vi "Launch Subordinate.vi"(6 "Position":T1, 8 "error in":errorcluster, 9 "Panel Definiton":T3, 10 "Identifier":string, 11 "Base Software in":refnum<class "Base Software.lvclass">) -> (0 "error out":errorcluster, 2 "Subordinate":T2, 3 "Base Software out":refnum<class "Base Software.lvclass">)   [LabVIEW 2019, in "Base Software.lvlib" / "Main.lvlib" / "Base Software.lvclass"]
uses:
  Project/Base Software.lvclass
  builds/Engine/Panel Manager.lvlibp/Panel Actor/Panel Actor.lvclass
  C:/Users/Public/Documents/Development/builds/Engine/Monitored Actor.lvlibp/Monitored Actor/Monitored Actor/Monitored Actor.lvclass
  builds/Engine/Panel.lvlibp/Panel/Panel.lvclass
  Custom Controls/Subordinate.ctl
  builds/Engine/Actor Framework.lvlibp/1abvi3w/vi.lib/ActorFramework/Message Enqueuer/Message Enqueuer.lvclass
  Custom Controls/Panel_Positions.ctl
  C:/Users/Public/Documents/Development/builds/Engine/Panel Manager.lvlibp/Panel Actor/Panel Actor.lvclass
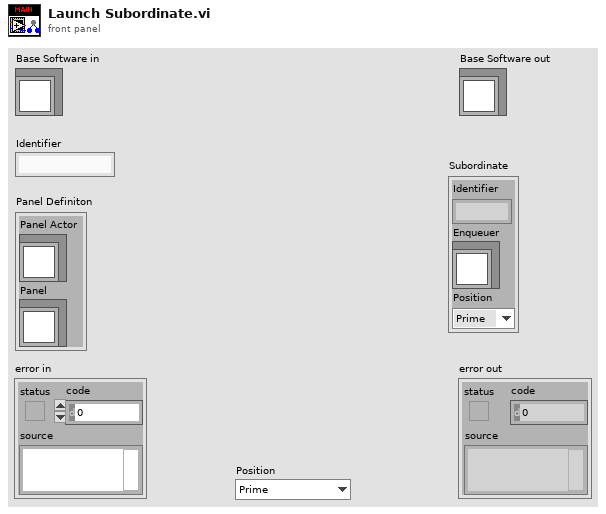
[diagram p1: front panel]
types:
  T1 = typedef "Base Software.lvlib/Main.lvlib/Base Software.lvclass/Panel_Positions.ctl" = enum16{"Prime", "Right", "Bottom", "Left", "Mission"}
  T2 = typedef "Base Software.lvlib/Main.lvlib/Base Software.lvclass/Subordinate.ctl" = cluster{"Identifier":string, "Enqueuer":refnum<class "Message Enqueuer.lvclass">, "Position":T1}
  T3 = cluster{"Panel Actor":refnum<class "Panel Actor.lvclass">, "Panel":refnum<class "Panel.lvclass">}
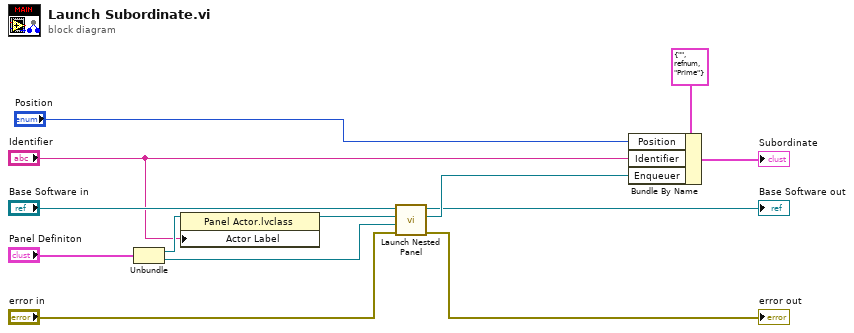
[diagram p0: block diagram]
diagram:
  n1 = Unbundle("Panel Definiton") -> ("Panel Actor"=w7:refnum<class "Panel Actor.lvclass">, "Panel"=w4:refnum<class "Panel.lvclass">)
  n2 = property class="Panel Actor.lvclass"(reference=w7, "Actor Label"="Identifier") -> (reference out=w6:refnum<class "Panel Actor.lvclass">)  [unwired: 1 in, 1 out]
  n3 = call "Launch Nested Panel.vi"("error in (no error)"="error in", "Panel"=w4, "Nested Panel Actor"=w6, "Panel Actor in"="Base Software in") -> ("error out"=→"error out":errorcluster, "Nested Actor's Enqueuer"=w12:refnum<class "Message Enqueuer.lvclass">, "Panel Actor out"=→"Base Software out":refnum<class "Base Software.lvclass">)  [unwired: 4 in, 1 out]
  n4 = Bundle By Name(cluster=T2 {"Identifier"="", "Enqueuer"=refnum, "Position"=enum."Prime"} ("Subordinate"), "Position"="Position", "Identifier"="Identifier", "Enqueuer"=w12) -> (→"Subordinate":T2)
